vi "Get Level.vi"(6 "Output Channel":T1, 8 "error in (no error)":errorcluster, 11 "RP100 in":refnum<class "RP100.lvclass">) -> (0 "error out":errorcluster, 2 "Level (V)":dbl, 3 "RP100 out":refnum<class "RP100.lvclass">)   [LabVIEW 2019, in "RP100.lvclass"]
uses:
  RP100.lvclass
  Typedefs/Output Channel--Enum.ctl
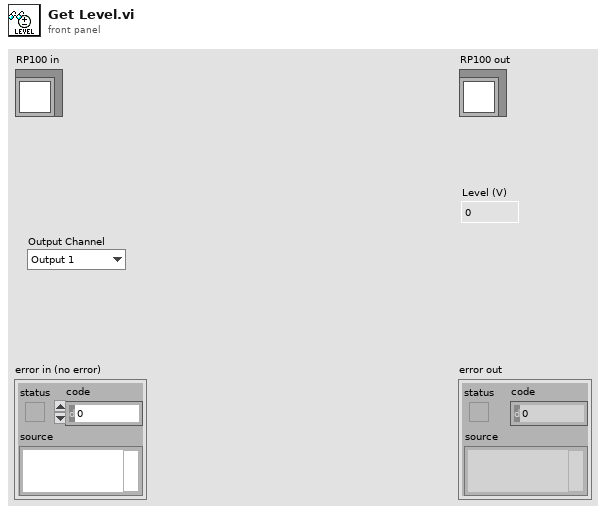
[diagram p1: front panel]
types:
  T1 = typedef "RP100.lvclass/Output Channel--Enum.ctl" = enum16{"Output 1", "Output 2"}
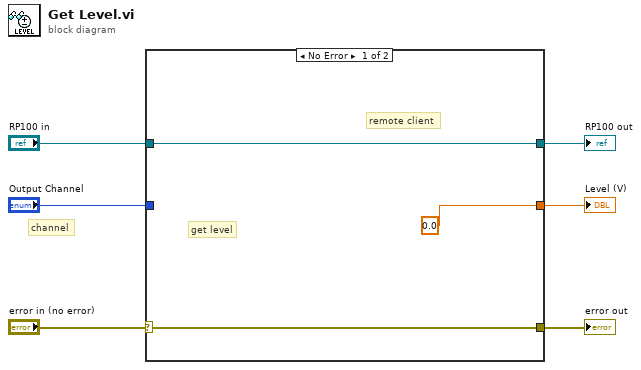
[diagram p0: block diagram]
diagram:
  # "channel"
  n1 = case shown="No Error" "error in (no error)" {
    selector: "error in (no error)" -> [w9 w11]
    tunnel: [w9 w11] -> w5
    tunnel: "RP100 in" -> [w8 w10]
    tunnel: [w8 w10] -> w3
    tunnel: [0.0 _] -> w1
    tunnel: "Output Channel" -> [_ _]
    frame No Error {
      # "remote client"
      # "get level"
    }
    frame Error {
    }
  }
  "error out" <- w5
  "RP100 out" <- w3
  "Level (V)" <- w1
